vi "Add Copyright.vi"() -> ()   [LabVIEW 2016]
doc: "A wrapper engine for adding/updating copyright text for LabVIEW files in a folder."
uses:
  SLL Tools/Copyright/_Typedefs/Select File Type.ctl
  <vilib>/Utility/error.llb/DialogType.ctl
  SLL Queued State Machine/Queue Driver/Create Queue.vi
  SLL Queued State Machine/Queue Driver/Enqueue an Item to Queue.vi
  SLL Queued State Machine/Queue Driver/Dequeue Queue.vi
  SLL Queued State Machine/Queue Driver/Enqueue N Items.vi
  SLL Queued State Machine/Queue Driver/Flush Queue.vi
  SLL Queued State Machine/Queue Driver/Release Queue.vi
  SLL Queued State Machine/SLL QSM.lvlib
  SLL Tools/Copyright/SLL Add Copyright.lvlib
panel:
  out "Progress":i32(slide) scale=0.0..10.0
  in  "Type":T1={"vi"=TRUE, "ctl"=TRUE, "lvlib"=TRUE, "lvclass"=TRUE, "lvproj"=TRUE} caption="Select File Type to Add Copyright"
  in  "Copyright Text":string="© Company Name"
  in  "Source Code Directory":path
  out "Status":string
  in  "Run":bool
  # "Add Copyright"
  # "Adds/updates copyright text to LabVIEW Files (VIs, Controls, Libraries, Classes and Projects)"
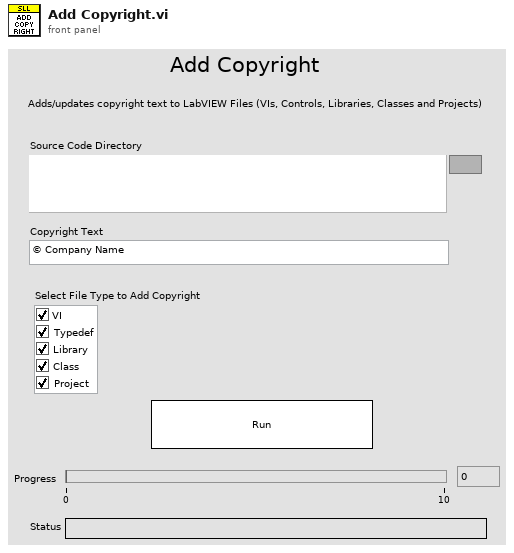
[diagram p1: front panel]
types:
  T1 = typedef "SLL Add Copyright.lvlib/Select File Type.ctl" = cluster{"vi":bool, "ctl":bool, "lvlib":bool, "lvclass":bool, "lvproj":bool}
  T2 = typedef "DialogType.ctl" = u16
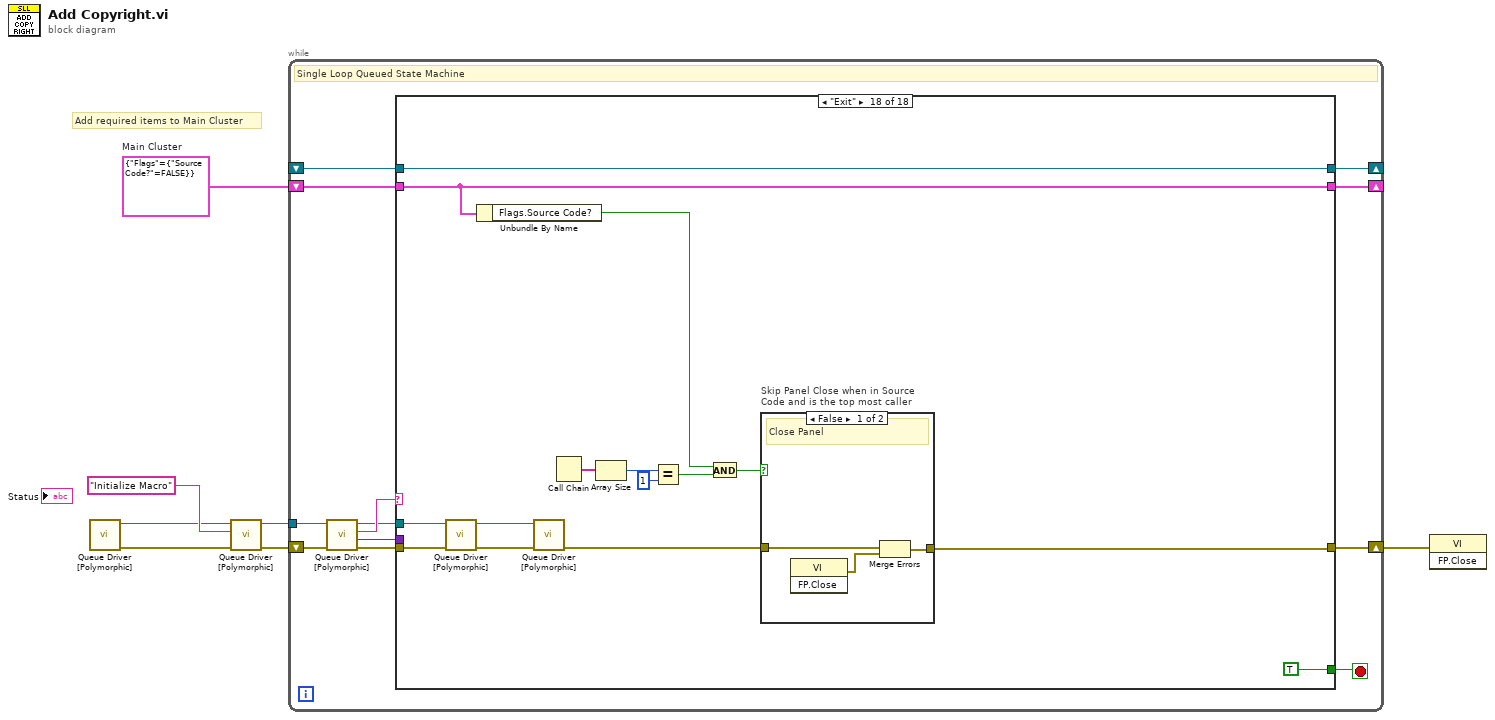
[diagram p0: block diagram]
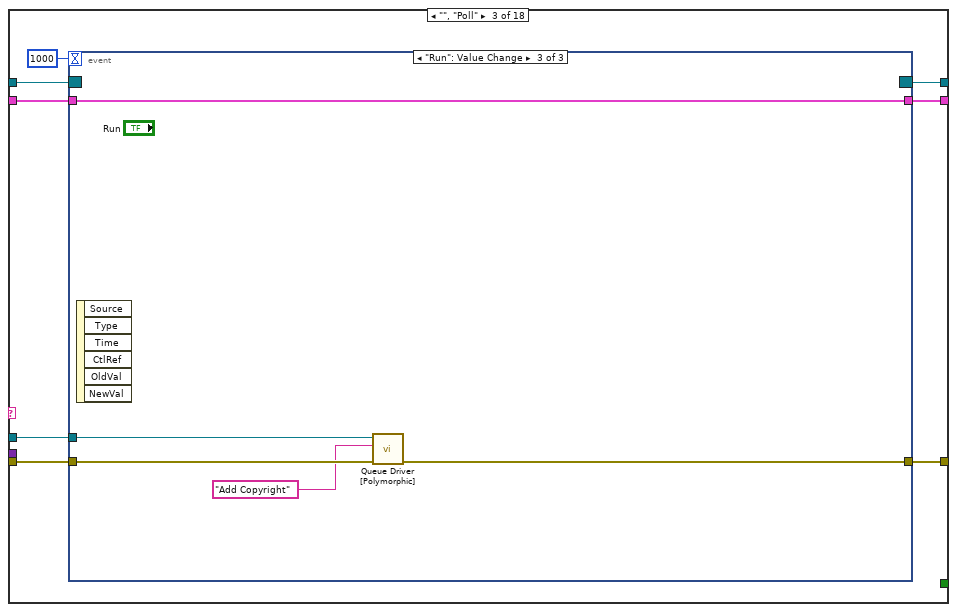
[diagram p4: hidden frame]
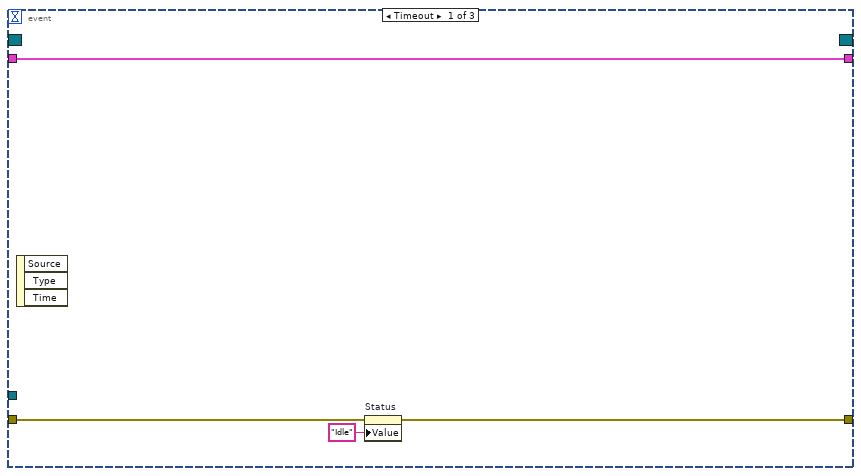
[diagram p5: hidden frame]
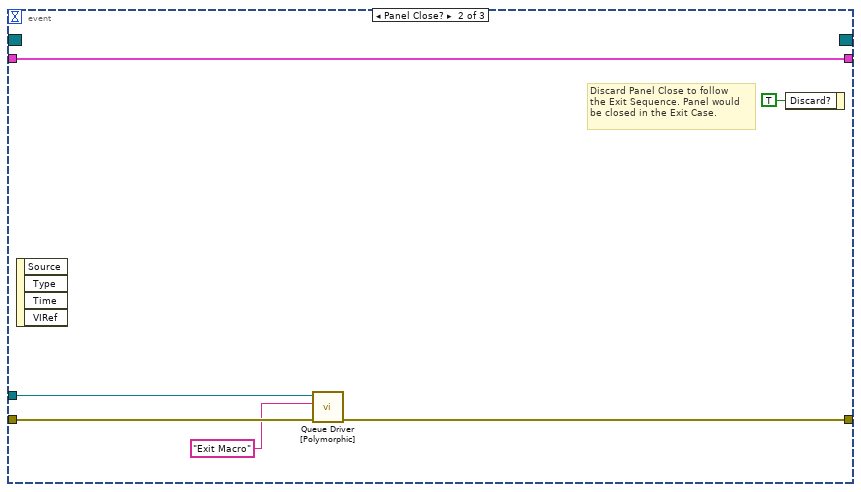
[diagram p6: hidden frame]
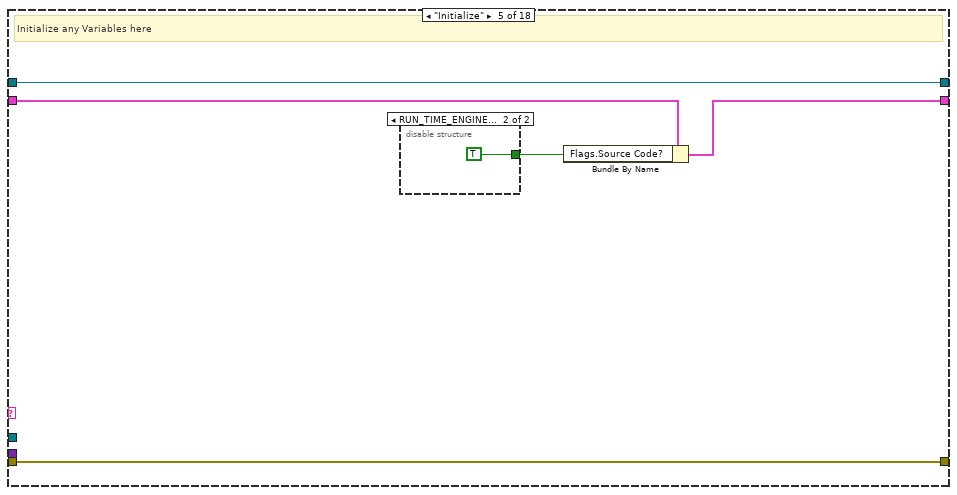
[diagram p8: hidden frame]
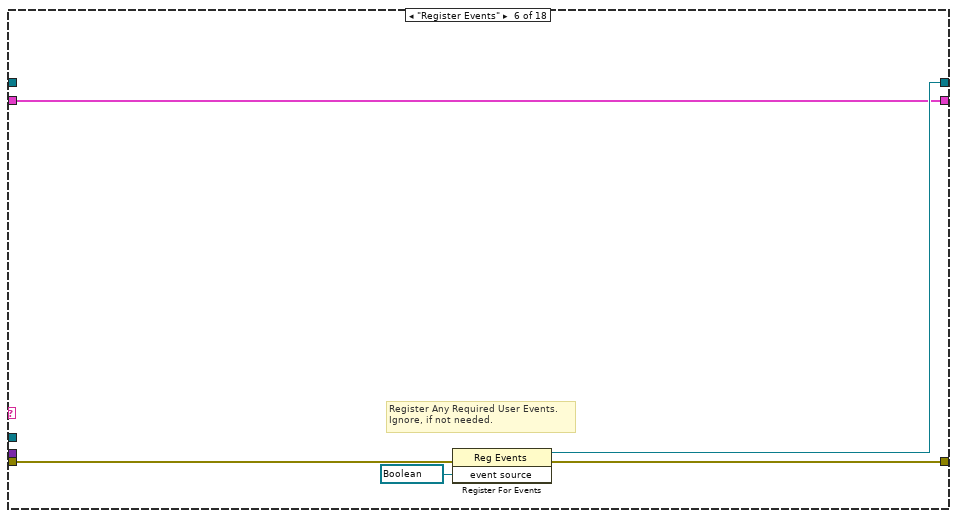
[diagram p10: hidden frame]
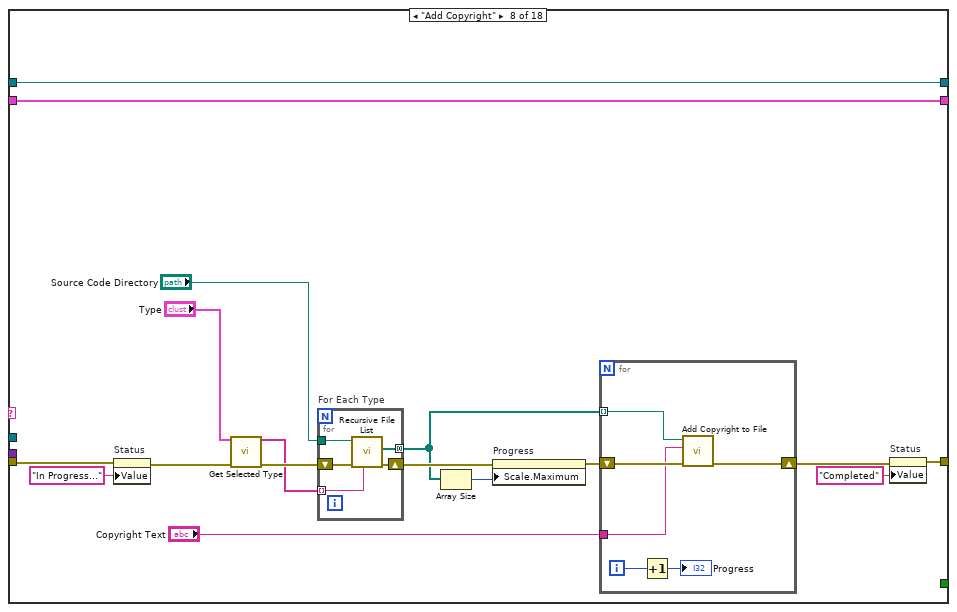
[diagram p12: hidden frame]
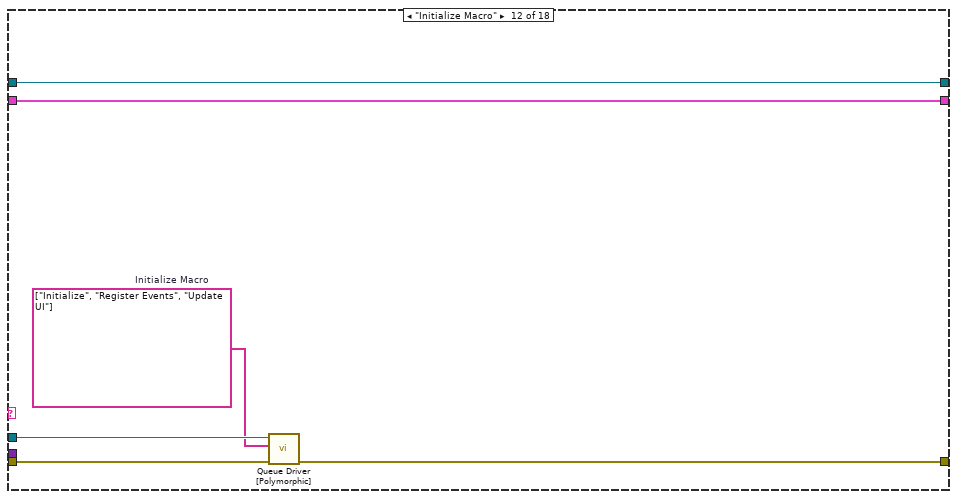
[diagram p16: hidden frame]
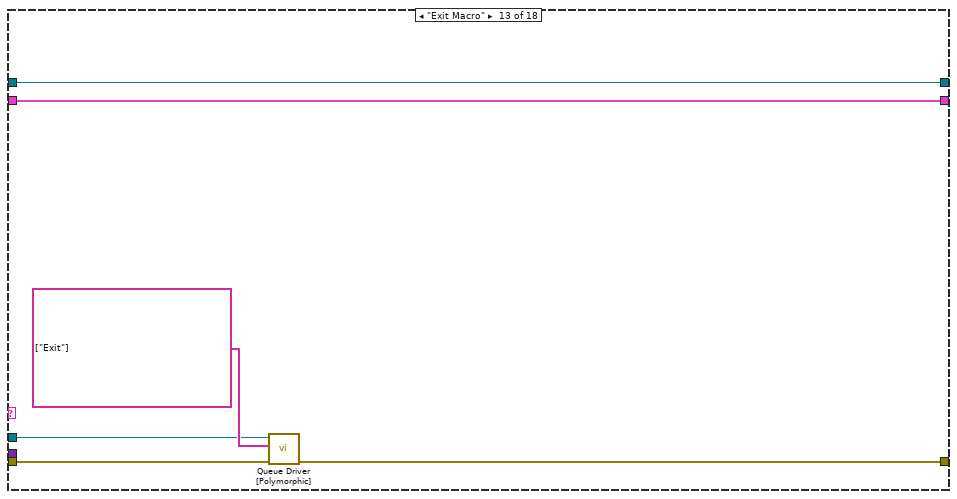
[diagram p17: hidden frame]
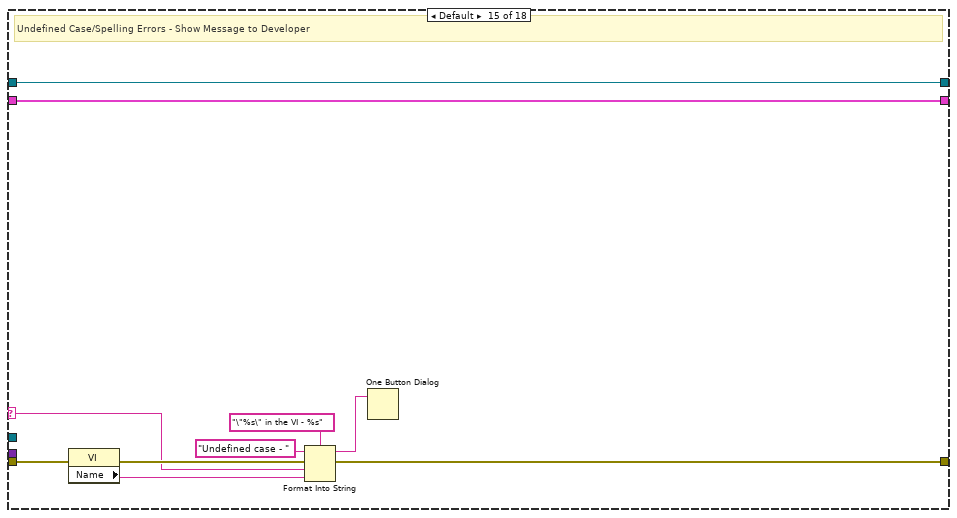
[diagram p19: hidden frame]
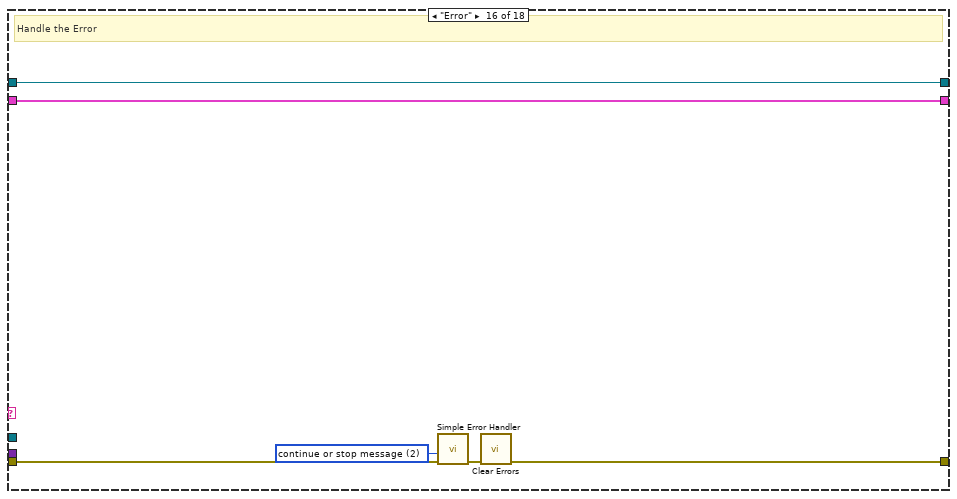
[diagram p20: hidden frame]
diagram:
  w5 = cluster{"Flags":cluster{"Source Code?":bool}} {"Flags"={"Source Code?"=FALSE}}  # Main Cluster
  # "Add required items to Main Cluster"
  n1 = call-poly "Queue Driver [Polymorphic].vi"() -> ("Error Out"=w7:errorcluster, "Queue Ref"=w3:refnum<queue>)  [unwired: 10 in]
  n2 = call-poly "Queue Driver [Polymorphic].vi"("Error In"=w7, "Item to Add"="Initialize Macro", "Queue Ref In"=w3) -> ("Error Out"=w6:errorcluster, "Queue Ref Out"=w2:refnum<queue>)  [unwired: 7 in]
  n3 = while "SLL Queued State Machine" {
    shift-right: [w17] -> w1
    shift-left: w6 -> [w19]
    shift-right: [w15] -> _
    shift-left: _ -> [w14]
    shift-right: [w13] -> _
    shift-left: w5 -> [w12]
    tunnel: w2 -> [w10]
    stop <- w16 stop-if-true
    # "Single Loop Queued State Machine"
    n4 = call-poly "Queue Driver [Polymorphic].vi"("Error In"=w19, "Queue Ref In"=w10) -> ("Error Out"=w18:errorcluster, "Data"=w8:variant, "Dequeue"=w11:string, "Queue Ref Out"=w9:refnum<queue>)  [unwired: 6 in]
    n5 = case "QSM Case Structure" shown="\"Exit\"" w11 {
      selector: w11 -> [_ _ _ _ _ _ _ _ _ _ _ _ _ _ w118 _ _ _]
      tunnel: w18 -> [w22 w25 w31 w51 w56 w62 w65 w80 w96 w99 w102 w106 w112 w117 w121 w133 w136 w149]
      tunnel: [w22 w25 w32 w51 w56 w61 w65 w78 w96 w99 w102 w105 w111 w117 w124 w131 w136 w145] -> w17
      tunnel: [_ _ _ _ _ _ _ _ _ _ _ _ _ _ _ _ _ TRUE] -> w16
      tunnel: [w21 w24 w30 w50 w55 w60 w64 w82 w95 w98 w101 w108 w114 w116 w127 w130 w135 w148] -> w15
      tunnel: w14 -> [w21 w24 w29 w50 w55 _ w64 w82 w95 w98 w101 w108 w114 w116 w127 w130 w135 w148]
      tunnel: [w20 w23 w27 w49 w52 w59 w63 w81 w94 w97 w100 w107 w113 w115 w126 w129 w134 w147] -> w13
      tunnel: w12 -> [w20 w23 w28 w49 w53 w59 w63 w81 w94 w97 w100 w107 w113 w115 w126 w129 w134 w147]
      tunnel: w9 -> [_ _ w26 _ _ _ _ _ _ _ _ w104 w109 _ _ _ _ w138]
      tunnel: w8 -> [_ _ _ _ _ _ _ _ _ _ _ _ _ _ _ _ _ _]
      frame "/--------------- Read Me -----------------/" {
        # "General Purpose Queue Based State Machine for Any Use Case (main application, module, pop up message etc)\n\nAdvantages:\n1. No Need to Pass Queue References between Queue Driver VIs.\n2. This template can be safely used in multiple parallel running modules without any issues.\n3. This template can also be safely used even in cases where the VI is configured to be a Clone, where multiple \ninstances of the VI could be executing concurrently.\n\nHow to Use:\n1. Add necessary items to the Main Cluster.\n2. Use the Polymorphic Queue Driver for doing any queue operations. There is no need to pass the queue driver\nreference, as the Queue Driver automatically infers the reference based on the VI instance from which it is called.\n3. Add any required user events in the \"Register Events\" case. Ignore if not needed.\n4. Use \"Sequences\" section for defining any list of state calls, which could be used in multiple places. \nExample: Initialize Sequence, might be needed if we need to any reinitialization."
      }
      frame "/------------------ Poll -------------------/" {
      }
      frame "", "Poll" {
        n6 = event shown="[2] \"Run\": Value Change" {
          selector: w29 -> [_ _ _]
          dyn-events: [_ _ _] -> w30
          timeout: 1000 -> [_ _ _]
          tunnel: [w34 w42 w47] -> w32
          tunnel: w31 -> [w35 w43 w48]
          tunnel: w28 -> [w37 w41 w46]
          tunnel: [w37 w41 w46] -> w27
          tunnel: w26 -> [_ w38 w44]
          event Timeout {
            n7 = event-data() -> ()  [unwired: 1 in, 3 out]
            n8 = property on="Status" class="Str"(error in=w35, "Value"="Idle" ("Status")) -> (error out=w34:errorcluster)  [unwired: 1 in, 1 out]
          }
          event Panel Close? {
            # "Discard Panel Close to follow\nthe Exit Sequence. Panel would\nbe closed in the Exit Case."
            n9 = event-data() -> ()  [unwired: 1 in, 4 out]
            n10 = call-poly "Queue Driver [Polymorphic].vi"("Error In"=w43, "Item to Add"="Exit Macro" ("Enqueue"), "Queue Ref In"=w38) -> ("Error Out"=w42:errorcluster)  [unwired: 7 in, 1 out]
            n11 = event-data("Discard?"=TRUE) -> ()  [unwired: 1 in, 1 out]
          }
          event "Run": Value Change {
            n12 = event-data() -> ()  [unwired: 1 in, 6 out]
            n13 = call-poly "Queue Driver [Polymorphic].vi"("Error In"=w48, "Item to Add"="Add Copyright" ("Enqueue"), "Queue Ref In"=w44) -> ("Error Out"=w47:errorcluster)  [unwired: 7 in, 1 out]
          }
        }
      }
      frame "/--------------- Initialize -----------------/" {
      }
      frame "Initialize" {
        # "Initialize any Variables here"
        n14 = disable-structure shown="RUN_TIME_ENGINE==False" {
          disable-tunnel: [_ TRUE] -> w54
          frame condition #0 {
          }
          frame condition #1 (active) {
          }
        }
        n15 = Bundle By Name(cluster=w53, "Flags.Source Code?"=w54) -> (w52:cluster{"Flags":cluster{"Source Code?":bool}})
      }
      frame "Register Events" {
        # "Register Any Required User Events. \nIgnore, if not needed."
        n16 = register-events(error in=w62, refnum<vi> refnum ("event source")) -> (reference out=w60:refnum<event-registration>, error out=w61:errorcluster)  [unwired: 1 in]
      }
      frame "/---------- Custom Case Splitter ----------/" {
      }
      frame "Add Copyright" {
        n17 = property on="Status" class="Str"(error in=w80, "Value"="In Progress..." ("Status")) -> (error out=w69:errorcluster)  [unwired: 1 in, 1 out]
        n18 = call "Get Selected Type.vi"("Select Type"="Type", "error in (no error)"=w69) -> ("Selected File Types[]"=w73:string[], "error out"=w75:errorcluster)  [unwired: 12 in]
        n19 = for "For Each Type" {
          tunnel: "Source Code Directory" -> [w85]
          tunnel: w73 -> [w84] mode=indexing
          tunnel: [w83] -> w72 mode=concatenating
          shift-right: [w86] -> w74
          shift-left: w75 -> [w87]
          n20 = call <vilib>:"Recursive File List.vi"("pattern"=w84, "error in (no error)"=w87, "Folder Path"=w85) -> ("error out"=w86:errorcluster, "All Files in Dir"=w83:path[])  [unwired: 4 in, 3 out]
        }
        n21 = Array Size(array=w72) -> (size(s)=w71:i32)
        n22 = property on="Progress" class="Slide (strict)"(error in=w74, "Scale.Maximum"=w71) -> (error out=w76:errorcluster)  [unwired: 1 in, 1 out]
        n23 = for {
          shift-right: [w91] -> w70
          shift-left: w76 -> [w92]
          tunnel: w72 -> [w93] mode=indexing
          tunnel: "Copyright Text" -> [w88]
          i -> [w90]
          n24 = Increment(x=w90) -> (x+1=→"Progress":i32)
          n25 = call "Add Copyright to File.vi"("error in (no error)"=w92, "Copyright Text"=w88, "File Path"=w93) -> ("error out"=w91:errorcluster)  [unwired: 8 in]
        }
        n26 = property on="Status" class="Str"(error in=w70, "Value"="Completed" ("Status")) -> (error out=w78:errorcluster)  [unwired: 1 in, 1 out]
      }
      frame "/-------------- User Interface --------------/" {
        # "Duplicate this case to create additional case splitters for readability"
      }
      frame "Update UI" {
        # "Update Front Panel Controls in this Case"
      }
      frame "/----------------- Macros -----------------/" {
      }
      frame "Initialize Macro" {
        w103 = string[] ["Initialize", "Register Events", "Update UI"]  # Initialize Macro
        n27 = call-poly "Queue Driver [Polymorphic].vi"("Error In"=w106, "Enqueue N"=w103, "Queue Ref In"=w104) -> ("Error Out"=w105:errorcluster)  [unwired: 7 in, 1 out]
      }
      frame "Exit Macro" {
        n28 = call-poly "Queue Driver [Polymorphic].vi"("Error In"=w112, "Enqueue N"=string[] ["Exit"], "Queue Ref In"=w109) -> ("Error Out"=w111:errorcluster)  [unwired: 7 in, 1 out]
      }
      frame "/-------------- Error Handler--------------/" {
      }
      frame Default {
        # "Undefined Case/Spelling Errors - Show Message to Developer"
        n29 = property class="VI"(error in=w121) -> (error out=w120:errorcluster, "Name"=w119:string)  [unwired: 1 in, 1 out]
        n30 = Format Into String(format string="\"%s\" in the VI - %s" ("message"), initial string="Undefined case - ", error in=w120, w118, w119) -> (resulting string=w122:string, error out=w124:errorcluster)
        n31 = One Button Dialog(message=w122) -> ()  [unwired: 1 in, 1 out]
      }
      frame "Error" {
        w128 = T2 2 items=["no dialog", "OK message", "continue or stop message", "OK message + warnings", "continue/stop + warnings"] ("type of dialog (OK msg:1)")
        # "Handle the Error"
        n32 = call <vilib>:"Simple Error Handler.vi"("type of dialog (OK msg:1)"=w128, "error in (no error)"=w133) -> ("error out"=w132:errorcluster)  [unwired: 3 in, 4 out]
        n33 = call <vilib>:"Clear Errors.vi"("error in (no error)"=w132) -> ("error out"=w131:errorcluster)  [unwired: 5 in, 1 out]
      }
      frame "/------------------- Exit --------------------/" {
      }
      frame "Exit" {
        n34 = call-poly "Queue Driver [Polymorphic].vi"("Error In"=w149, "Queue Ref In"=w138) -> ("Error Out"=w150:errorcluster, "Queue Ref Out"=w137:refnum<queue>)  [unwired: 7 in, 1 out]
        n35 = Unbundle By Name(w147) -> ("Flags.Source Code?"=w140:bool)
        n36 = call-poly "Queue Driver [Polymorphic].vi"("Error In"=w150, "Queue Ref In"=w137) -> ("Error Out"=w146:errorcluster)  [unwired: 9 in]
        n37 = Call Chain() -> (call chain=w144:string[])
        n38 = Array Size(array=w144) -> (size(s)=w143:i32)
        n39 = Equal?(x=w143, y=1) -> (x = y?=w141:bool)
        n40 = And(x=w140, y=w141) -> (x .and. y?=w139:bool)
        n41 = case "Skip Panel Close when in Source\nCode and is the top most caller" shown="False" w139 {
          tunnel: w146 -> [w153 w155]
          tunnel: [w154 w155] -> w145
          frame False {
            # "Close Panel"
            n42 = invoke class="VI" method="FP.Close"() -> (error out=w152:errorcluster)  [unwired: 3 in, 2 out]
            n43 = Merge Errors(w153, w152) -> (w154:errorcluster)
          }
          frame True {
            # "Do Not Close Panel"
          }
        }
      }
    }
  }
  n44 = invoke class="VI" method="FP.Close"(error in=w1) -> ()  [unwired: 2 in, 3 out]
